vi "修改操作.vi"(1 "VI输入":refnum<vi>, 3 "修改控件名称":string, 4 "错误输入（无错误）":errorcluster, 6 "修改后控件名称":string, 7 "修改控件类型":T1(ring)) -> (0 "错误输出":errorcluster)   [LabVIEW 2018]
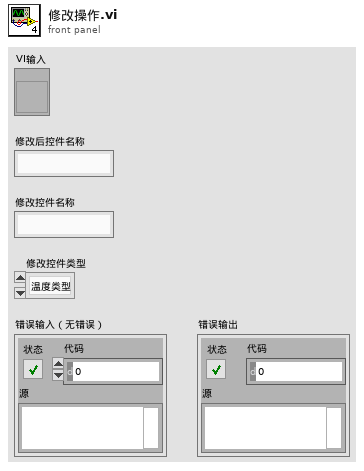
[diagram p1: front panel]
types:
  T1 = enum16{"温度类型", "压力类型", "压差类型", "流量类型", "液位类型", "电流类型", "电压类型", "调节阀", "开关阀"}
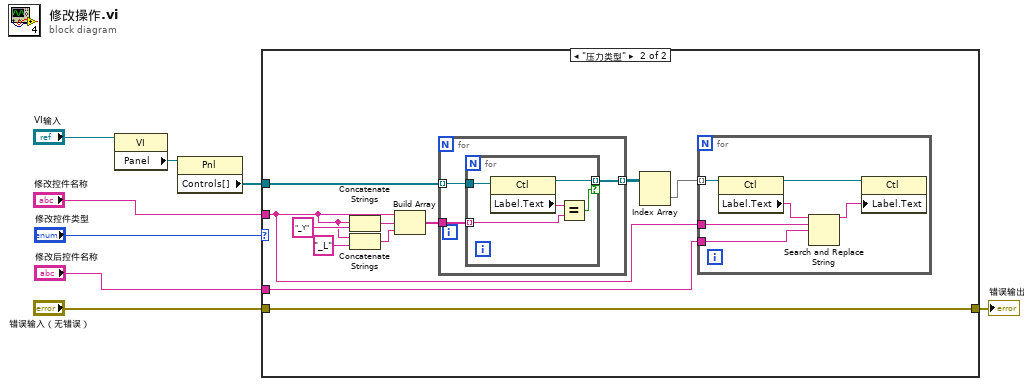
[diagram p0: block diagram]
diagram:
  n1 = property class="VI"(reference="VI输入") -> ("Panel"=w2:refnum<vi>)  [unwired: 1 in, 2 out]
  n2 = property class="Pnl"(reference=w2) -> ("Controls[]"=w4:refnum<vi>[])  [unwired: 1 in, 2 out]
  n3 = case shown="\"压力类型\"" "修改控件类型" {
    tunnel: "修改控件名称" -> [_ w12]
    tunnel: w4 -> [_ w20]
    tunnel: "错误输入（无错误）" -> [w9 w19]
    tunnel: [w9 w19] -> w7
    tunnel: "修改后控件名称" -> [_ w11]
    frame "温度类型", Default {
    }
    frame "压力类型" {
      n4 = Concatenate Strings(w12, "_Y" ("字符串")) -> (w17:string)
      n5 = Concatenate Strings(w12, "_L" ("字符串")) -> (w15:string)
      n6 = Build Array(w12, w17, w15) -> (w18:string[])
      n7 = for {
        tunnel: w18 -> [w29]
        tunnel: w20 -> [w28] mode=indexing
        tunnel: [w27] -> w13 mode=indexing
        n8 = for {
          tunnel: w29 -> [w32] mode=indexing
          tunnel: w28 -> [w34]
          tunnel: [w31] -> w27 mode=indexing if=w30
          n9 = property class="Ctl"(reference=w34) -> (reference out=w31:refnum<vi>, "Label.Text"=w33:string)  [unwired: 1 in, 1 out]
          n10 = Equal?(x=w33, y=w32) -> (x = y?=w30:bool)
        }
      }
      n11 = Index Array(array=w13) -> (element=w10:refnum<vi>[])  [unwired: 2 in]
      n12 = for {
        tunnel: w10 -> [w26] mode=indexing
        tunnel: w12 -> [w22]
        tunnel: w11 -> [w21]
        n13 = property class="Ctl"(reference=w26) -> (reference out=w25:refnum<vi>, "Label.Text"=w23:string)  [unwired: 1 in, 1 out]
        n14 = Search and Replace String(input string=w23, search string=w22, replace string=w21) -> (result string=w24:string)  [unwired: 5 in, 3 out]
        n15 = property class="Ctl"(reference=w25, "Label.Text"=w24) -> ()  [unwired: 1 in, 2 out]
      }
    }
  }
  "错误输出" <- w7
